vi "GENser Meas Output Current.vi"(7 "GEN Addr":i16=-1, 8 "error":errorcluster, 11 "VISA":refnum<visa-resource-name>) -> (0 "error out":errorcluster, 2 "Output Current":dbl format="%.4f", 3 "VISA out":refnum<visa-resource-name>)   [LabVIEW 2017]
doc: "This VI returns the output current, in amps, measured by the power supply.\n(query \"MC?\")"
panel:
  # "Lambda Genesys \nSerial Port\n  DC Power Supplies"
  # "Measure the \nOutput Current"
  # "-1 = no address change"
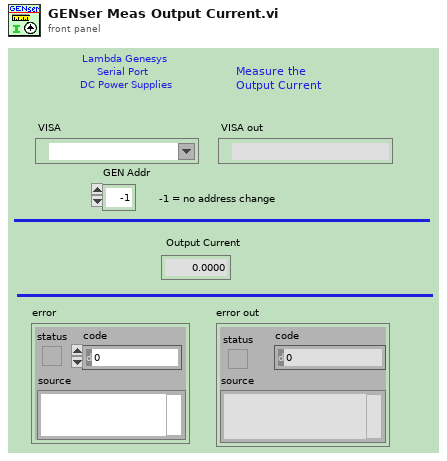
[diagram p1: front panel]
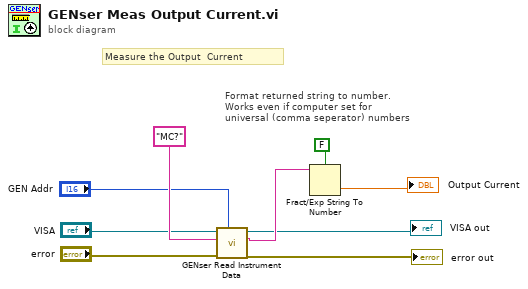
[diagram p0: block diagram]
diagram:
  # "Format returned string to number.\nWorks even if computer set for \nuniversal (comma seperator) numbers"
  # "Measure the Output  Current"
  n1 = call "GENser Read Instrument Data.vi"("GEN Addr"="GEN Addr", "error"="error", "Query"="MC?" ("format string"), "VISA"="VISA") -> ("error out"=→"error out":errorcluster, "Response"=w7:string, "VISA out"=→"VISA out":refnum<visa-resource-name>)  [unwired: 4 in, 1 out]
  n2 = Fract/Exp String To Number(use system decimal point (T)=FALSE, string=w7) -> (number=→"Output Current":dbl)  [unwired: 2 in, 1 out]
